vi "chart_bar.vi"() -> ()   [LabVIEW 8.6]
uses:
  Controls/lxw_chart_type.ctl
  Controls/lxw_chart_axis_type.ctl
  Controls/style_id.ctl
panel:
  out "error out":errorcluster
  out "function return 2":string
  # "chart_bar.xlsx"
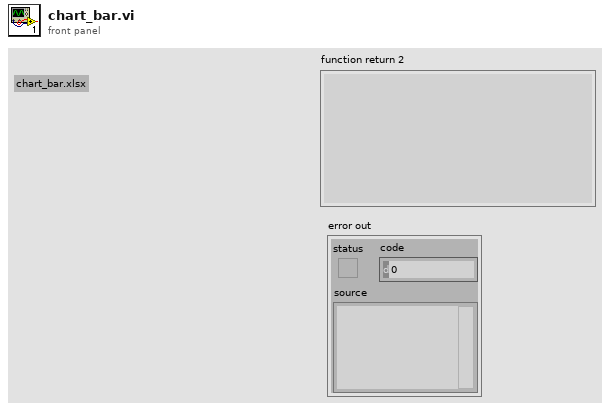
[diagram p1: front panel]
types:
  T1 = typedef "style_id.ctl" = u16
  T2 = typedef "lxw_chart_axis_type.ctl" = u8
  T3 = typedef "lxw_chart_type.ctl" = u8
  T4 = enum32{"invalid app kind", "Development System", "Run Time System", "Student Edition", "Embedded LabVIEW", "Evaluation", "Custom"}
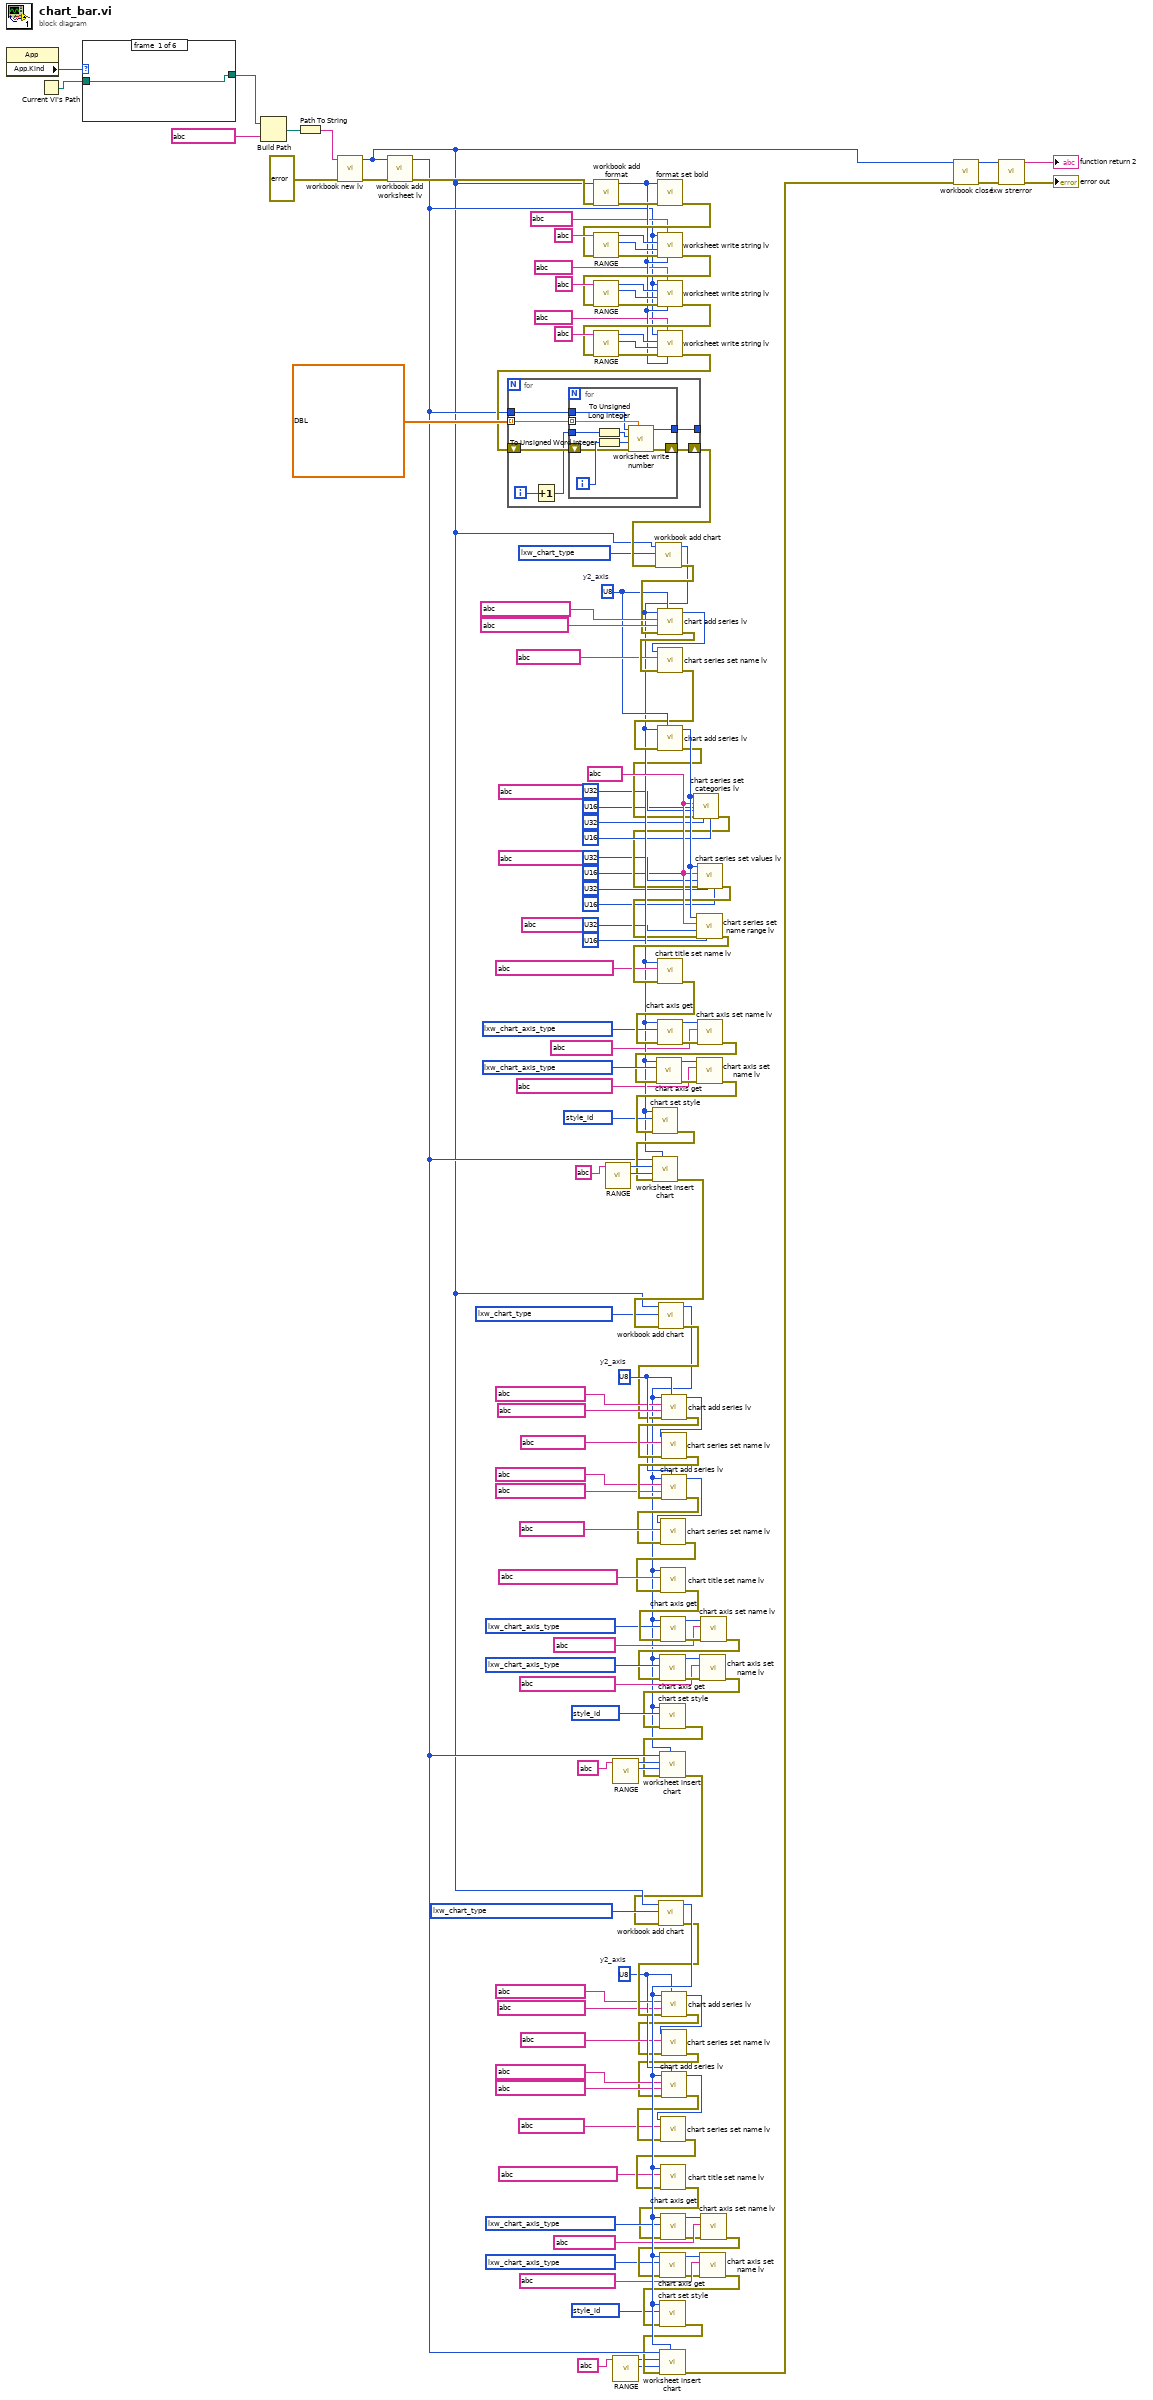
[diagram p0: block diagram]
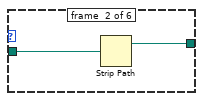
[diagram p2: hidden frame]
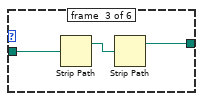
[diagram p3: hidden frame]
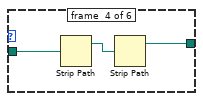
[diagram p4: hidden frame]
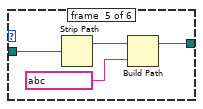
[diagram p5: hidden frame]
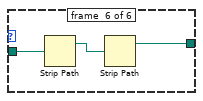
[diagram p6: hidden frame]
diagram:
  w31 = T1 ? items=["Style_1", "Style_2", "Style_3", "Style_4", "Style_5", "Style_6", "Style_7", "Style_8", "Style_9", "Style_10", "Style_11", "Style_12", "Style_13", "Style_14", "Style_15", "Style_16", "Style_17", "Style_18", "Style_19", "Style_20", "Style_21", "Style_22", "Style_23", "Style_24", "Style_25", "Style_26", "Style_27", "Style_28", "Style_29", "Style_30", "Style_31", "Style_32", "Style_33", "Style_34", "Style_35", "Style_36", "Style_37", "Style_38", "Style_39", "Style_40", "Style_41", "Style_42", "Style_43", "Style_44", "Style_45", "Style_46", "Style_47", "Style_48"] ("style_id")
  w23 = T2 ? items=["LXW_CHART_AXIS_TYPE_X", "LXW_CHART_AXIS_TYPE_Y", "LXW_CHART_AXIS_TYPE_X2", "LXW_CHART_AXIS_TYPE_Y2"] ("axis_type")
  w18 = T2 ? items=["LXW_CHART_AXIS_TYPE_X", "LXW_CHART_AXIS_TYPE_Y", "LXW_CHART_AXIS_TYPE_X2", "LXW_CHART_AXIS_TYPE_Y2"] ("axis_type")
  w7 = u8 ?  # y2_axis
  w2 = T3 ? items=["LXW_CHART_NONE", "LXW_CHART_AREA", "LXW_CHART_AREA_STACKED", "LXW_CHART_AREA_STACKED_PERCENT", "LXW_CHART_BAR", "LXW_CHART_BAR_STACKED", "LXW_CHART_BAR_STACKED_PERCENT", "LXW_CHART_COLUMN", "LXW_CHART_COLUMN_STACKED", "LXW_CHART_COLUMN_STACKED_PERCENT", "LXW_CHART_DOUGHNUT", "LXW_CHART_LINE", "LXW_CHART_LINE_STACKED", "LXW_CHART_LINE_STACKED_PERCENT", "LXW_CHART_PIE", "LXW_CHART_SCATTER", "LXW_CHART_SCATTER_STRAIGHT", "LXW_CHART_SCATTER_STRAIGHT_WITH_MARKERS", "LXW_CHART_SCATTER_SMOOTH", "LXW_CHART_SCATTER_SMOOTH_WITH_MARKERS", "LXW_CHART_RADAR", "LXW_CHART_RADAR_WITH_MARKERS", "LXW_CHART_RADAR_FILLED", "LXW_CHART_STOCK"] ("chart_type")
  w38 = T1 ? items=["Style_1", "Style_2", "Style_3", "Style_4", "Style_5", "Style_6", "Style_7", "Style_8", "Style_9", "Style_10", "Style_11", "Style_12", "Style_13", "Style_14", "Style_15", "Style_16", "Style_17", "Style_18", "Style_19", "Style_20", "Style_21", "Style_22", "Style_23", "Style_24", "Style_25", "Style_26", "Style_27", "Style_28", "Style_29", "Style_30", "Style_31", "Style_32", "Style_33", "Style_34", "Style_35", "Style_36", "Style_37", "Style_38", "Style_39", "Style_40", "Style_41", "Style_42", "Style_43", "Style_44", "Style_45", "Style_46", "Style_47", "Style_48"] ("style_id")
  w46 = T2 ? items=["LXW_CHART_AXIS_TYPE_X", "LXW_CHART_AXIS_TYPE_Y", "LXW_CHART_AXIS_TYPE_X2", "LXW_CHART_AXIS_TYPE_Y2"] ("axis_type")
  w51 = T2 ? items=["LXW_CHART_AXIS_TYPE_X", "LXW_CHART_AXIS_TYPE_Y", "LXW_CHART_AXIS_TYPE_X2", "LXW_CHART_AXIS_TYPE_Y2"] ("axis_type")
  w62 = u8 ?  # y2_axis
  w67 = T3 ? items=["LXW_CHART_NONE", "LXW_CHART_AREA", "LXW_CHART_AREA_STACKED", "LXW_CHART_AREA_STACKED_PERCENT", "LXW_CHART_BAR", "LXW_CHART_BAR_STACKED", "LXW_CHART_BAR_STACKED_PERCENT", "LXW_CHART_COLUMN", "LXW_CHART_COLUMN_STACKED", "LXW_CHART_COLUMN_STACKED_PERCENT", "LXW_CHART_DOUGHNUT", "LXW_CHART_LINE", "LXW_CHART_LINE_STACKED", "LXW_CHART_LINE_STACKED_PERCENT", "LXW_CHART_PIE", "LXW_CHART_SCATTER", "LXW_CHART_SCATTER_STRAIGHT", "LXW_CHART_SCATTER_STRAIGHT_WITH_MARKERS", "LXW_CHART_SCATTER_SMOOTH", "LXW_CHART_SCATTER_SMOOTH_WITH_MARKERS", "LXW_CHART_RADAR", "LXW_CHART_RADAR_WITH_MARKERS", "LXW_CHART_RADAR_FILLED", "LXW_CHART_STOCK"] ("chart_type")
  w88 = T1 ? items=["Style_1", "Style_2", "Style_3", "Style_4", "Style_5", "Style_6", "Style_7", "Style_8", "Style_9", "Style_10", "Style_11", "Style_12", "Style_13", "Style_14", "Style_15", "Style_16", "Style_17", "Style_18", "Style_19", "Style_20", "Style_21", "Style_22", "Style_23", "Style_24", "Style_25", "Style_26", "Style_27", "Style_28", "Style_29", "Style_30", "Style_31", "Style_32", "Style_33", "Style_34", "Style_35", "Style_36", "Style_37", "Style_38", "Style_39", "Style_40", "Style_41", "Style_42", "Style_43", "Style_44", "Style_45", "Style_46", "Style_47", "Style_48"] ("style_id")
  w94 = T2 ? items=["LXW_CHART_AXIS_TYPE_X", "LXW_CHART_AXIS_TYPE_Y", "LXW_CHART_AXIS_TYPE_X2", "LXW_CHART_AXIS_TYPE_Y2"] ("axis_type")
  w99 = T2 ? items=["LXW_CHART_AXIS_TYPE_X", "LXW_CHART_AXIS_TYPE_Y", "LXW_CHART_AXIS_TYPE_X2", "LXW_CHART_AXIS_TYPE_Y2"] ("axis_type")
  (unwired) string ? ("range_str")
  (unwired) string ? ("range_str")
  (unwired) string ? ("range_str")
  w102 = string ? ("sheetname")
  w107 = u8 ?  # y2_axis
  w113 = T3 ? items=["LXW_CHART_NONE", "LXW_CHART_AREA", "LXW_CHART_AREA_STACKED", "LXW_CHART_AREA_STACKED_PERCENT", "LXW_CHART_BAR", "LXW_CHART_BAR_STACKED", "LXW_CHART_BAR_STACKED_PERCENT", "LXW_CHART_COLUMN", "LXW_CHART_COLUMN_STACKED", "LXW_CHART_COLUMN_STACKED_PERCENT", "LXW_CHART_DOUGHNUT", "LXW_CHART_LINE", "LXW_CHART_LINE_STACKED", "LXW_CHART_LINE_STACKED_PERCENT", "LXW_CHART_PIE", "LXW_CHART_SCATTER", "LXW_CHART_SCATTER_STRAIGHT", "LXW_CHART_SCATTER_STRAIGHT_WITH_MARKERS", "LXW_CHART_SCATTER_SMOOTH", "LXW_CHART_SCATTER_SMOOTH_WITH_MARKERS", "LXW_CHART_RADAR", "LXW_CHART_RADAR_WITH_MARKERS", "LXW_CHART_RADAR_FILLED", "LXW_CHART_STOCK"] ("chart_type")
  n1 = property class="App"() -> ("App.Kind"=w150:T4)  [unwired: 2 in, 2 out]
  n2 = Current VI's Path() -> (path=w149:path)
  n3 = case shown="\"Evaluation\"" w150 {
    tunnel: w149 -> [w151 w153 w156 w159 w163 w166]
    tunnel: [w151 w152 w154 w157 w161 w164] -> w148
    frame #0 {
    }
    frame #1 {
      n4 = Strip Path(path=w153) -> (stripped path=w152:path)  [unwired: 1 out]
    }
    frame #2 {
      n5 = Strip Path(path=w156) -> (stripped path=w155:path)  [unwired: 1 out]
      n6 = Strip Path(path=w155) -> (stripped path=w154:path)  [unwired: 1 out]
    }
    frame #3 {
      n7 = Strip Path(path=w159) -> (stripped path=w158:path)  [unwired: 1 out]
      n8 = Strip Path(path=w158) -> (stripped path=w157:path)  [unwired: 1 out]
    }
    frame #4 {
      n9 = Strip Path(path=w163) -> (stripped path=w162:path)  [unwired: 1 out]
      n10 = Build Path(base path=w162, name or relative path=string ?) -> (appended path=w161:path)
    }
    frame #5 {
      n11 = Strip Path(path=w166) -> (stripped path=w165:path)  [unwired: 1 out]
      n12 = Strip Path(path=w165) -> (stripped path=w164:path)  [unwired: 1 out]
    }
  }
  n13 = Build Path(base path=w148, name or relative path=string ? ("filename")) -> (appended path=w140:path)
  n14 = Path To String(path=w140) -> (string=w139:string)
  n15 = call "workbook new lv.vi"("error in (no error)"=errorcluster ?, "filename"=w139) -> ("error out"=w146:errorcluster, "function return"=w82:u32)  [unwired: 8 in]
  n16 = call "workbook add worksheet lv.vi"("error in (no error)"=w146, "workbook"=w82) -> ("error out"=w118:errorcluster, "function return"=w83:u32)  [unwired: 8 in]
  n17 = call "workbook add format.vi"("error in (no error)"=w118, "workbook"=w82) -> ("error out"=w123:errorcluster, "function return"=w121:u32)  [unwired: 8 in]
  n18 = call "RANGE.vi"("range_str"=string ?) -> ("col"=w91:u16, "row"=w90:u32)  [unwired: 6 in, 3 out]
  n19 = call "RANGE.vi"("range_str"=string ?) -> ("col"=w41:u16, "row"=w40:u32)  [unwired: 6 in, 3 out]
  n20 = call "RANGE.vi"("range_str"=string ?) -> ("col"=w28:u16, "row"=w29:u32)  [unwired: 6 in, 3 out]
  n21 = call "format set bold.vi"("error in (no error)"=w123, "format"=w121) -> ("error out"=w122:errorcluster)  [unwired: 9 in]
  n22 = call "RANGE.vi"("error in (no error)"=w122, "range_str"=string ?) -> ("error out"=w134:errorcluster, "col"=w130:u16, "row"=w131:u32)  [unwired: 5 in, 2 out]
  n23 = call "worksheet write string lv.vi"("format"=w121, "string"=string ?, "error in (no error)"=w134, "col"=w130, "row"=w131, "worksheet"=w83) -> ("error out"=w125:errorcluster)  [unwired: 4 in, 1 out]
  n24 = call "RANGE.vi"("error in (no error)"=w125, "range_str"=string ?) -> ("error out"=w133:errorcluster, "col"=w128:u16, "row"=w129:u32)  [unwired: 5 in, 2 out]
  n25 = call "worksheet write string lv.vi"("format"=w121, "string"=string ?, "error in (no error)"=w133, "col"=w128, "row"=w129, "worksheet"=w83) -> ("error out"=w124:errorcluster)  [unwired: 4 in, 1 out]
  n26 = call "RANGE.vi"("error in (no error)"=w124, "range_str"=string ?) -> ("error out"=w132:errorcluster, "col"=w126:u16, "row"=w127:u32)  [unwired: 5 in, 2 out]
  n27 = call "worksheet write string lv.vi"("format"=w121, "string"=string ?, "error in (no error)"=w132, "col"=w126, "row"=w127, "worksheet"=w83) -> ("error out"=w119:errorcluster)  [unwired: 4 in, 1 out]
  n28 = for {
    tunnel: dbl[][] ? -> [w173] mode=indexing
    shift-right: [w171] -> w120
    shift-left: w119 -> [w172]
    tunnel: w83 -> [w170]
    tunnel: [w169] -> _
    i -> [w168]
    n29 = Increment(x=w168) -> (x+1=w167:i32)
    n30 = for {
      tunnel: w173 -> [w182] mode=indexing
      tunnel: w167 -> [w179]
      shift-right: [w176] -> w171
      shift-left: w172 -> [w177]
      tunnel: w170 -> [w175]
      tunnel: [w174] -> w169
      i -> [w181]
      n31 = To Unsigned Long Integer(number=w179) -> (unsigned 32bit integer=w178:u32)
      n32 = To Unsigned Word Integer(number=w181) -> (unsigned 16bit integer=w180:u16)
      n33 = call "worksheet write number.vi"("number"=w182, "error in (no error)"=w177, "col"=w180, "row"=w178, "worksheet"=w175) -> ("error out"=w176:errorcluster, "function return"=w174:u32)  [unwired: 5 in]
    }
  }
  n34 = call "workbook add chart.vi"("error in (no error)"=w120, "chart_type"=w113, "workbook"=w82) -> ("error out"=w108:errorcluster, "function return"=w86:u32)  [unwired: 7 in]
  n35 = call "chart add series lv.vi"("y2_axis"=w107, "error in (no error)"=w108, "values"=string ?, "categories"=string ?, "chart"=w86) -> ("error out"=w112:errorcluster, "function return"=w105:u32)  [unwired: 5 in]
  n36 = call "chart series set name lv.vi"("error in (no error)"=w112, "name"=string ? ("values"), "series"=w105) -> ("error out"=w106:errorcluster)  [unwired: 8 in]
  n37 = call "chart add series lv.vi"("y2_axis"=w107, "error in (no error)"=w106, "chart"=w86) -> ("error out"=w80:errorcluster, "function return"=w104:u32)  [unwired: 7 in]
  n38 = call "chart series set categories lv.vi"("last_col"=u16 ?, "last_row"=u32 ?, "first_col"=u16 ?, "error in (no error)"=w80, "first_row"=u32 ?, "sheetname"=w102, "series"=w104) -> ("error out"=w75:errorcluster)  [unwired: 4 in]
  n39 = call "chart series set values lv.vi"("last_col"=u16 ?, "last_row"=u32 ?, "first_col"=u16 ?, "error in (no error)"=w75, "first_row"=u32 ?, "sheetname"=w102, "series"=w104) -> ("error out"=w74:errorcluster)  [unwired: 4 in]
  n40 = call "chart series set name range lv.vi"("col"=u16 ?, "error in (no error)"=w74, "row"=u32 ?, "sheetname"=w102, "series"=w104) -> ("error out"=w103:errorcluster)  [unwired: 6 in]
  n41 = call "chart title set name lv.vi"("error in (no error)"=w103, "name"=string ?, "chart"=w86) -> ("error out"=w100:errorcluster)  [unwired: 8 in]
  n42 = call "chart axis get.vi"("error in (no error)"=w100, "axis_type"=w99, "chart"=w86) -> ("error out"=w97:errorcluster, "function return"=w98:u32)  [unwired: 7 in]
  n43 = call "chart axis set name lv.vi"("error in (no error)"=w97, "name"=string ?, "axis"=w98) -> ("error out"=w93:errorcluster)  [unwired: 8 in]
  n44 = call "chart axis get.vi"("error in (no error)"=w93, "axis_type"=w94, "chart"=w86) -> ("error out"=w96:errorcluster, "function return"=w95:u32)  [unwired: 7 in]
  n45 = call "chart axis set name lv.vi"("error in (no error)"=w96, "name"=string ?, "axis"=w95) -> ("error out"=w92:errorcluster)  [unwired: 8 in]
  n46 = call "chart set style.vi"("error in (no error)"=w92, "style_id"=w88, "chart"=w86) -> ("error out"=w87:errorcluster)  [unwired: 8 in]
  n47 = call "worksheet insert chart.vi"("chart"=w86, "error in (no error)"=w87, "col"=w91, "row"=w90, "worksheet"=w83) -> ("error out"=w114:errorcluster)  [unwired: 5 in, 1 out]
  n48 = call "workbook add chart.vi"("error in (no error)"=w114, "chart_type"=w67, "workbook"=w82) -> ("error out"=w60:errorcluster, "function return"=w35:u32)  [unwired: 7 in]
  n49 = call "chart add series lv.vi"("y2_axis"=w62, "error in (no error)"=w60, "values"=string ?, "categories"=string ?, "chart"=w35) -> ("error out"=w66:errorcluster, "function return"=w55:u32)  [unwired: 5 in]
  n50 = call "chart series set name lv.vi"("error in (no error)"=w66, "name"=string ? ("values"), "series"=w55) -> ("error out"=w65:errorcluster)  [unwired: 8 in]
  n51 = call "chart add series lv.vi"("y2_axis"=w62, "error in (no error)"=w65, "values"=string ?, "categories"=string ?, "chart"=w35) -> ("error out"=w56:errorcluster, "function return"=w54:u32)  [unwired: 5 in]
  n52 = call "chart series set name lv.vi"("error in (no error)"=w56, "name"=string ? ("values"), "series"=w54) -> ("error out"=w42:errorcluster)  [unwired: 8 in]
  n53 = call "chart title set name lv.vi"("error in (no error)"=w42, "name"=string ?, "chart"=w35) -> ("error out"=w52:errorcluster)  [unwired: 8 in]
  n54 = call "chart axis get.vi"("error in (no error)"=w52, "axis_type"=w51, "chart"=w35) -> ("error out"=w49:errorcluster, "function return"=w50:u32)  [unwired: 7 in]
  n55 = call "chart axis set name lv.vi"("error in (no error)"=w49, "name"=string ?, "axis"=w50) -> ("error out"=w45:errorcluster)  [unwired: 8 in]
  n56 = call "chart axis get.vi"("error in (no error)"=w45, "axis_type"=w46, "chart"=w35) -> ("error out"=w48:errorcluster, "function return"=w47:u32)  [unwired: 7 in]
  n57 = call "chart axis set name lv.vi"("error in (no error)"=w48, "name"=string ?, "axis"=w47) -> ("error out"=w36:errorcluster)  [unwired: 8 in]
  n58 = call "chart set style.vi"("error in (no error)"=w36, "style_id"=w38, "chart"=w35) -> ("error out"=w37:errorcluster)  [unwired: 8 in]
  n59 = call "worksheet insert chart.vi"("chart"=w35, "error in (no error)"=w37, "col"=w41, "row"=w40, "worksheet"=w83) -> ("error out"=w1:errorcluster)  [unwired: 5 in, 1 out]
  n60 = call "workbook add chart.vi"("error in (no error)"=w1, "chart_type"=w2, "workbook"=w82) -> ("error out"=w9:errorcluster, "function return"=w34:u32)  [unwired: 7 in]
  n61 = call "chart add series lv.vi"("y2_axis"=w7, "error in (no error)"=w9, "values"=string ?, "categories"=string ?, "chart"=w34) -> ("error out"=w3:errorcluster, "function return"=w14:u32)  [unwired: 5 in]
  n62 = call "chart series set name lv.vi"("error in (no error)"=w3, "name"=string ? ("values"), "series"=w14) -> ("error out"=w4:errorcluster)  [unwired: 8 in]
  n63 = call "chart add series lv.vi"("y2_axis"=w7, "error in (no error)"=w4, "values"=string ?, "categories"=string ?, "chart"=w34) -> ("error out"=w13:errorcluster, "function return"=w15:u32)  [unwired: 5 in]
  n64 = call "chart series set name lv.vi"("error in (no error)"=w13, "name"=string ? ("values"), "series"=w15) -> ("error out"=w27:errorcluster)  [unwired: 8 in]
  n65 = call "chart title set name lv.vi"("error in (no error)"=w27, "name"=string ?, "chart"=w34) -> ("error out"=w17:errorcluster)  [unwired: 8 in]
  n66 = call "chart axis get.vi"("error in (no error)"=w17, "axis_type"=w18, "chart"=w34) -> ("error out"=w20:errorcluster, "function return"=w19:u32)  [unwired: 7 in]
  n67 = call "chart axis set name lv.vi"("error in (no error)"=w20, "name"=string ?, "axis"=w19) -> ("error out"=w24:errorcluster)  [unwired: 8 in]
  n68 = call "chart axis get.vi"("error in (no error)"=w24, "axis_type"=w23, "chart"=w34) -> ("error out"=w21:errorcluster, "function return"=w22:u32)  [unwired: 7 in]
  n69 = call "chart axis set name lv.vi"("error in (no error)"=w21, "name"=string ?, "axis"=w22) -> ("error out"=w33:errorcluster)  [unwired: 8 in]
  n70 = call "chart set style.vi"("error in (no error)"=w33, "style_id"=w31, "chart"=w34) -> ("error out"=w32:errorcluster)  [unwired: 8 in]
  n71 = call "worksheet insert chart.vi"("chart"=w34, "error in (no error)"=w32, "col"=w28, "row"=w29, "worksheet"=w83) -> ("error out"=w81:errorcluster)  [unwired: 5 in, 1 out]
  n72 = call "workbook close.vi"("error in (no error)"=w81, "workbook"=w82) -> ("error out"=w142:errorcluster, "function return"=w144:u32)  [unwired: 8 in]
  n73 = call "lxw strerror.vi"("error in (no error)"=w142, "error_num"=w144) -> ("error out"=→"error out":errorcluster, "function return"=→"function return 2":string)  [unwired: 8 in]
